vi "send_array_to_python_and_back.vi"() -> ()   [LabVIEW 2014]
panel:
  out "resulting string":string
  in  "milliseconds to wait":u32=300
  out "array":dbl[](array[numeric])
  out "python error out":string
  out "python output":string
  in  "# of points between python calls":i32=30
  out "XY Graph":cluster{"X":dbl[], "Y":dbl[]}[](graph)
  out "raw python input":dbl[][](array[numeric])
  in  "Stop Button":bool
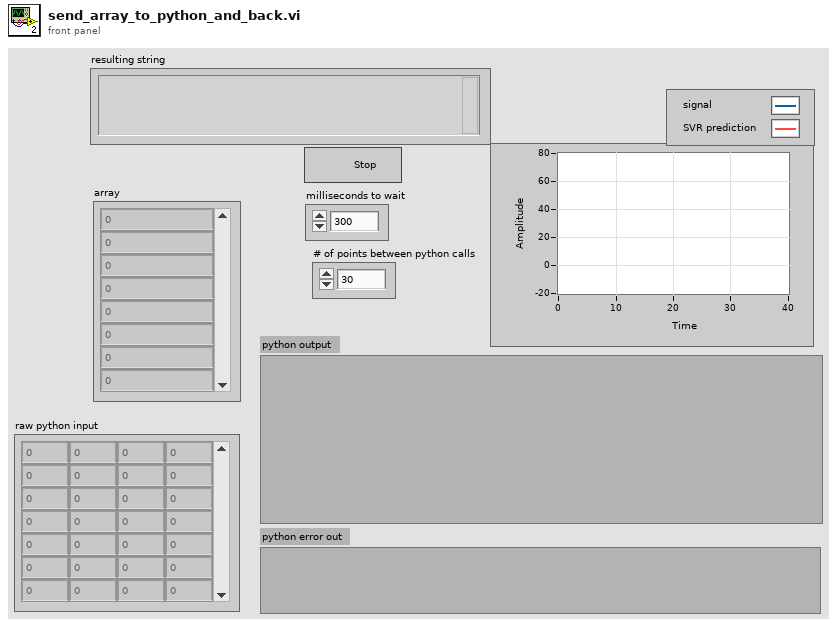
[diagram p1: front panel]
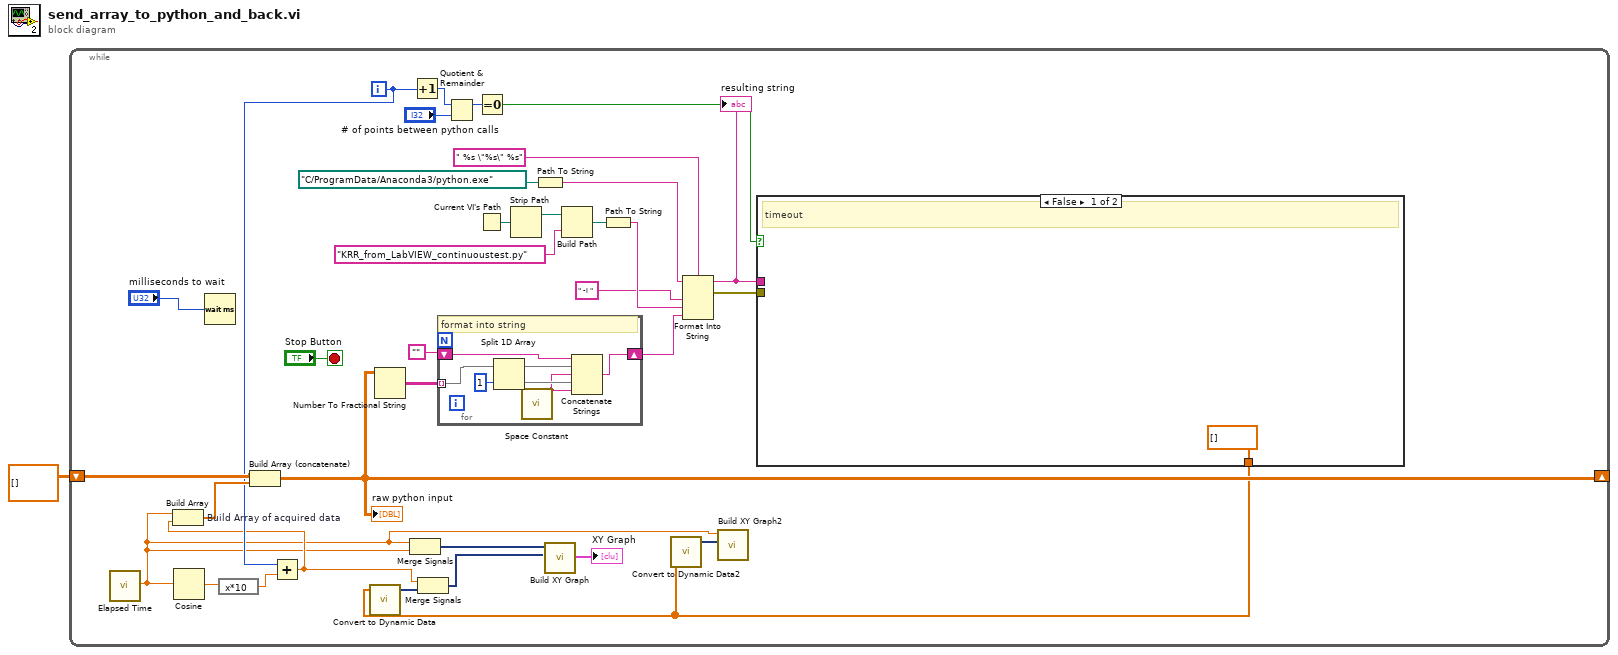
[diagram p0: block diagram]
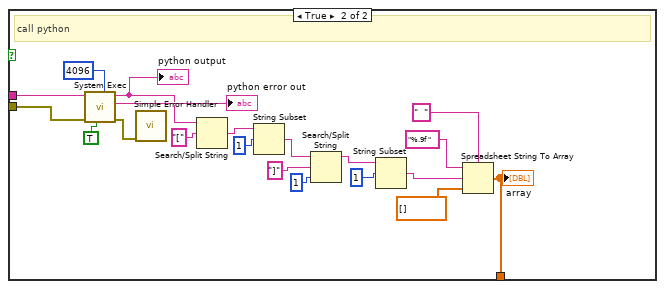
[diagram p2: hidden frame]
diagram:
  n1 = while {
    shift-right: [w26] -> _
    shift-left: dbl[][] [] -> [w33]
    i -> [w7]
    stop <- "Stop Button" stop-if-true
    n2 = call "Elapsed Time"() -> ("Elapsed Time (s)"=w3:dbl)  [unwired: 12 in, 7 out]
    n3 = Cosine(x=w3) -> (cos(x)=w28:dbl)
    n4 = Wait (ms)(milliseconds to wait="milliseconds to wait") -> ()  [unwired: 1 out]
    n5 = expression code="x*10"(w28) -> (w6:dbl)
    n6 = Add(x=w7, y=w6) -> (x+y=w5:dbl)
    n7 = Build Array "Build Array of acquired data"(w3, w5) -> (w34:dbl[])
    n8 = Build Array (concatenate)(w33, w34) -> (w26:dbl[][])
    "raw python input" <- w26
    n9 = Number To Fractional String(number=w26) -> (F-format string=w16:string[][])  [unwired: 3 in]
    n10 = Merge Signals(w3, w3) -> (w11:dynamicdata)
    n11 = Increment(x=w7) -> (x+1=w30:i32)
    n12 = for {
      shift-right: [w40] -> w14
      shift-left: "" -> [w39]
      tunnel: w16 -> [w37] mode=indexing
      # "format into string"
      n13 = Split 1D Array(array=w37, index=1) -> (first subarray=w42:string[], second subarray=w41:string[])
      n14 = call <vilib>:"Space Constant.vi"() -> ("String"=w36:string)
      n15 = Concatenate Strings(w39, w42, w36, w41, w36) -> (w40:string)
    }
    n16 = Quotient & Remainder(x=w30, y="# of points between python calls") -> (x-y*floor(x/y)=w31:i32)  [unwired: 1 out]
    n17 = Equal To 0?(x=w31) -> (x = 0?=w29:bool)
    n18 = Current VI's Path() -> (path=w24:path)
    n19 = Strip Path(path=w24) -> (stripped path=w22:path)  [unwired: 1 out]
    n20 = Path To String(path=path "C:/ProgramData/Anaconda3/python.exe" ("Path to Python.exe")) -> (string=w20:string)
    n21 = Build Path(base path=w22, name or relative path="KRR_from_LabVIEW_continuoustest.py" ("Path to Function")) -> (appended path=w19:path)
    n22 = Path To String(path=w19) -> (string=w9:string)
    n23 = Format Into String(format string=" %s \"%s\" %s", initial string=w20, " -i " ("input 2"), w9, w14) -> (resulting string=w18:string, error out=w17:errorcluster)  [unwired: 1 in]
    "resulting string" <- w18
    n24 = case shown="False" w29 {
      tunnel: w18 -> [_ w60]
      tunnel: w17 -> [_ w59]
      tunnel: [dbl[] [] ("array type (2D Dbl)") w44] -> w2
      frame False {
        # "timeout"
      }
      frame True {
        # "call python"
        n25 = call <vilib>:"System Exec.vi"("expected output size  (4096)"=u32 4096, "run minimized? (F)"=TRUE, "error in (no error)"=w59, "command line"=w60) -> ("error out"=w61:errorcluster, "standard error"=→"python error out":string, "standard output"=w54:string)  [unwired: 4 in, 1 out]
        "python output" <- w54
        n26 = call <vilib>:"Simple Error Handler.vi"("error in (no error)"=w61) -> ()  [unwired: 4 in, 5 out]
        n27 = Search/Split String(string=w54, search string/char (-)="[") -> (match + rest of string=w53:string)  [unwired: 1 in, 2 out]
        n28 = String Subset(string=w53, offset (0)=1) -> (substring=w52:string)  [unwired: 1 in]
        n29 = Search/Split String(string=w52, search string/char (-)="]", offset (0)=1) -> (substring before match=w46:string)  [unwired: 2 out]
        n30 = String Subset(string=w46, offset (0)=1) -> (substring=w45:string)  [unwired: 1 in]
        n31 = Spreadsheet String To Array(delimiter (Tab)="  ", format string="%.9f ", spreadsheet string=w45, array type (2D Dbl)=dbl[] []) -> (array=w44:dbl[])
        "array" <- w44
      }
    }
    n32 = call "Convert to Dynamic Data"("Array"=w2) -> ("Dynamic Data Type"=w12:dynamicdata)  [unwired: 3 in]
    n33 = Merge Signals(w5, w12) -> (w13:dynamicdata)
    n34 = call "Build XY Graph"("Y Input"=w13, "X Input"=w11) -> ("XY Graph"=→"XY Graph":cluster{"X":dbl[], "Y":dbl[]}[])  [unwired: 8 in, 1 out]
    n35 = call "Convert to Dynamic Data2"("Array"=w2) -> ("Dynamic Data Type"=w4:dynamicdata)  [unwired: 3 in]
    n36 = call "Build XY Graph2"("Y Input"=w4, "X Input"=w3) -> ()  [unwired: 8 in, 2 out]
  }
